vi "Treat Command.vi"(8 "error in (no error)":errorcluster, 11 "Channel in":refnum<class "Channel.lvclass">) -> (0 "error out":errorcluster, 3 "Channel out":refnum<class "Channel.lvclass">)   [LabVIEW 2018, in "Channel.lvclass"]
doc: "Treat the commando received from the control interface."
uses:
  Channel.lvclass
  Channel.lvclass/Channel.ctl
  State Machine/CCS_State Machine.lvclass
  Simulated_CCD_Camera/Simulated Camera.lvclass
  RxTx/CCS_RxTx.lvclass
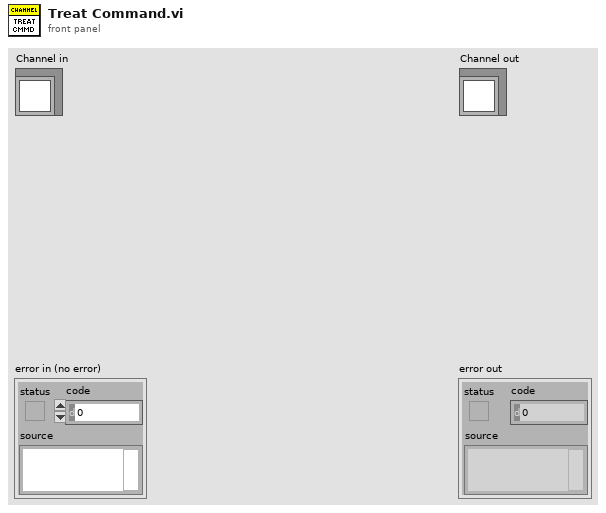
[diagram p1: front panel]
types:
  T1 = cluster{"CYCLES_DONE":u16, "LAST_IMAGE_NAME":string, "USED_DISK_SPACE":u16, "FRAMES_DONE":u16, "CCD_STATUS":string, "CURRENT_TEMPERATURE":i16, "TEMPERATURE_STATUS":string, "FRAME_EXPOSURE_TIME":sgl, "ERROR":bool, "SERIAL_NUMBER":u16, "ACQUIRING":bool, "IMAGE_INDEX":u32, "SEQS_DONE":u16}
  T2 = cluster{"COOLER_POWER_STATUS":u16, "TEMP":i32, "EXPTIME":dbl, "#FRAMES":u32, "#CYCLES":u32, "#SEQS":u32, "WAVEPLATE_POS":u16}
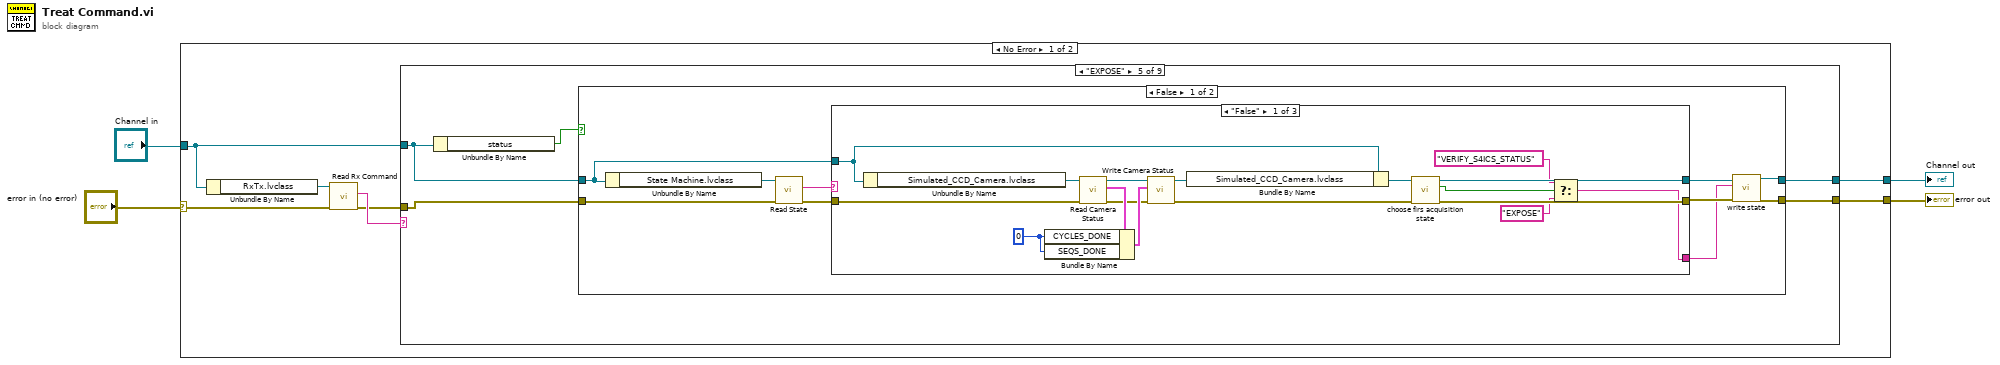
[diagram p0: block diagram]
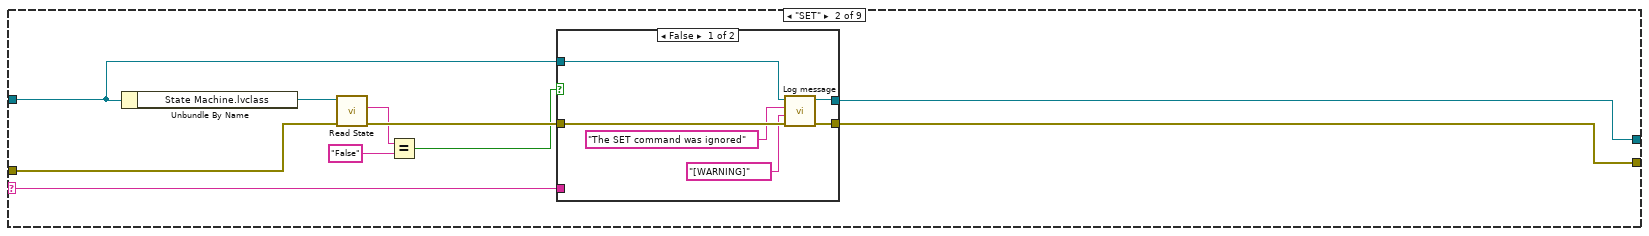
[diagram p3: hidden frame]
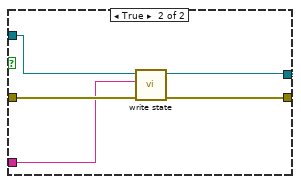
[diagram p4: hidden frame]
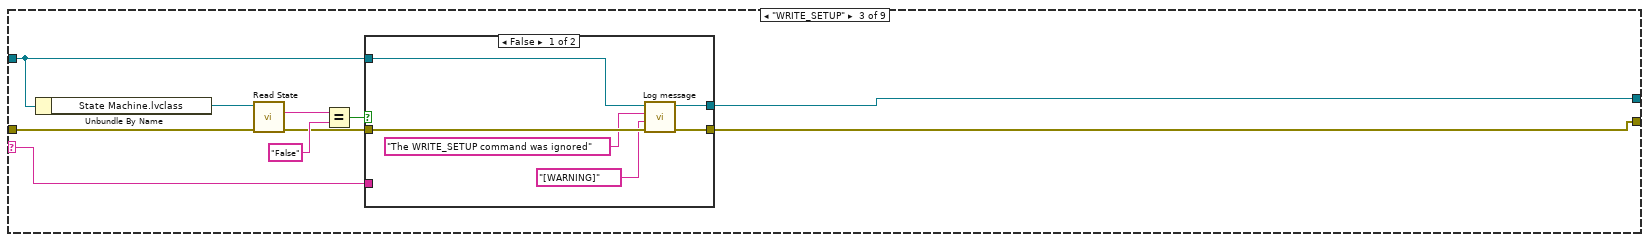
[diagram p5: hidden frame]
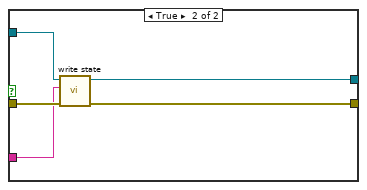
[diagram p6: hidden frame]
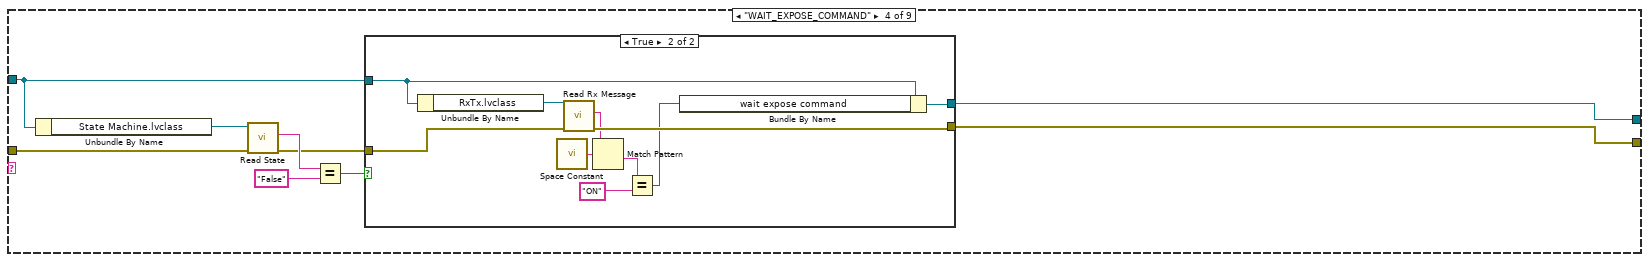
[diagram p7: hidden frame]
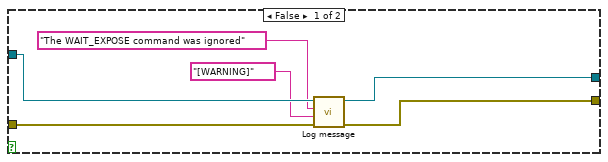
[diagram p8: hidden frame]
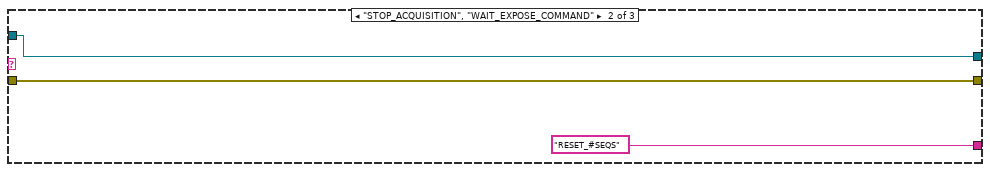
[diagram p9: hidden frame]
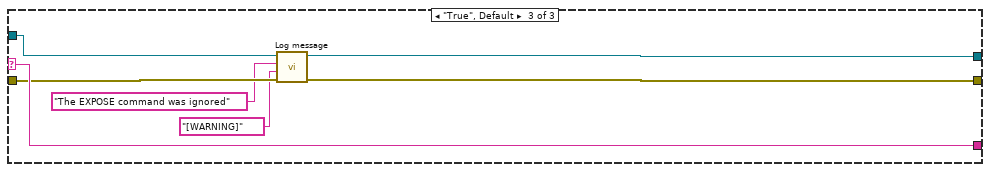
[diagram p10: hidden frame]
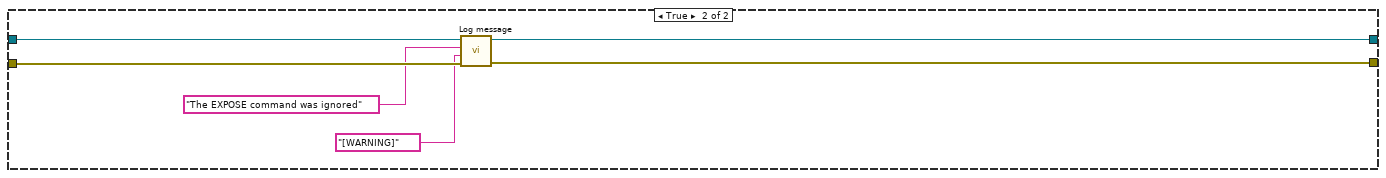
[diagram p11: hidden frame]
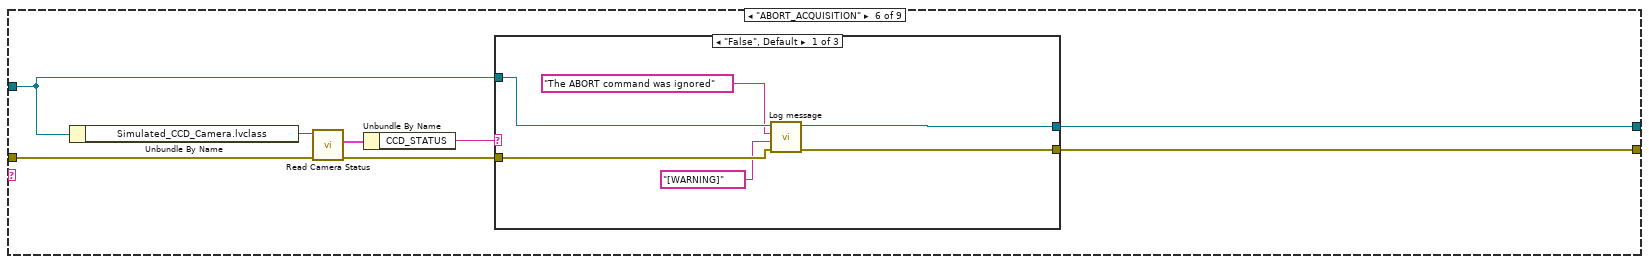
[diagram p12: hidden frame]
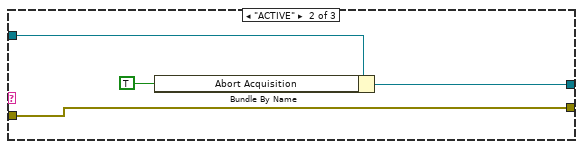
[diagram p13: hidden frame]
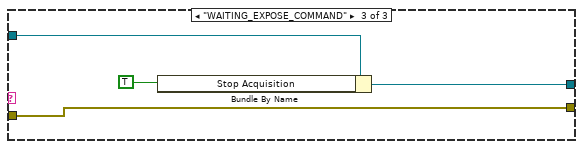
[diagram p14: hidden frame]
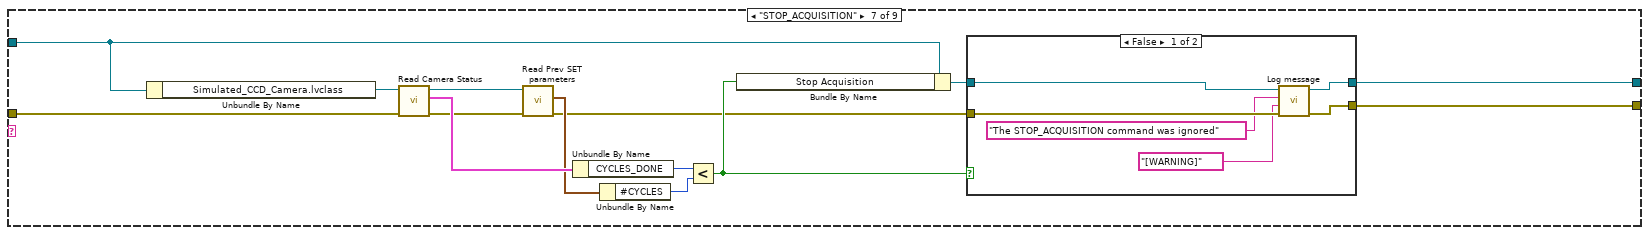
[diagram p15: hidden frame]
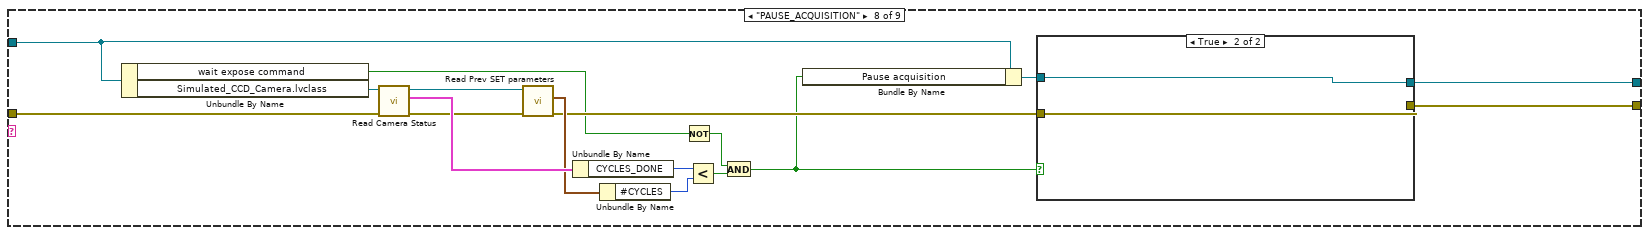
[diagram p17: hidden frame]
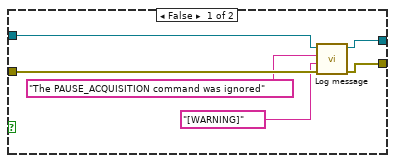
[diagram p18: hidden frame]
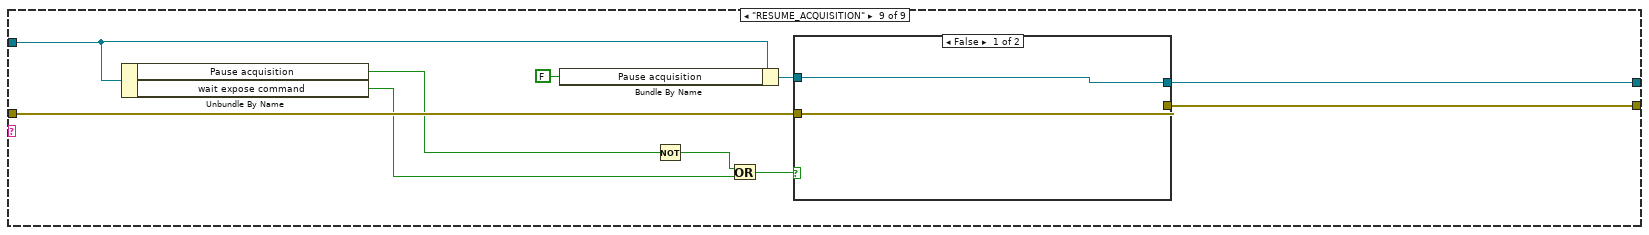
[diagram p19: hidden frame]
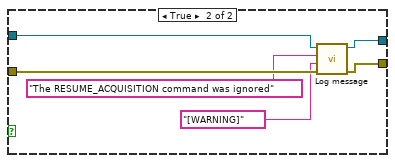
[diagram p20: hidden frame]
diagram:
  n1 = case shown="No Error" "error in (no error)" {
    selector: "error in (no error)" -> [w10 w217]
    tunnel: [w7 w217] -> w3
    tunnel: [w8 w216] -> w1
    tunnel: "Channel in" -> [w6 w216]
    frame No Error {
      n2 = Unbundle By Name(w6) -> ("RxTx.lvclass"=w11:refnum<class "CCS_RxTx.lvclass">)
      n3 = call "Read Rx Command.vi"("error in (no error)"=w10, "RxTx in"=w11) -> ("error out"=w5:errorcluster, "Rx Command"=w9:string)  [unwired: 7 in, 1 out]
      n4 = case shown="\"EXPOSE\"" w9 {
        selector: w9 -> [_ w15 w35 _ _ _ _ _ _]
        tunnel: w6 -> [w13 w17 w39 w59 w82 w136 w164 w189 w207]
        tunnel: [w13 w19 w38 w57 w84 w135 w152 w180 w205] -> w8
        tunnel: w5 -> [w12 w20 w42 w62 w83 w133 w158 w183 w206]
        tunnel: [w12 w18 w37 w56 w85 w129 w151 w179 w204] -> w7
        frame "False", Default {
        }
        frame "SET" {
          n5 = Unbundle By Name(w17) -> ("State Machine.lvclass"=w22:refnum<class "CCS_State Machine.lvclass">)
          n6 = call-dynamic "Read State.vi"("error in (no error)"=w20, "State Machine in"=w22) -> ("error out"=w23:errorcluster, "State"=w16:string)  [unwired: 7 in, 1 out]
          n7 = Equal?(x=w16, y="False") -> (x = y?=w14:bool)
          n8 = case shown="False" w14 {
            tunnel: w23 -> [w29 w31]
            tunnel: [w27 w33] -> w19
            tunnel: [w28 w32] -> w18
            tunnel: w17 -> [w26 w34]
            tunnel: w15 -> [_ w30]
            frame False {
              n9 = call "Log message.vi"("error in (no error)"=w29, "message type"="[WARNING]", "String"="The SET command was ignored", "Channel in"=w26) -> ("error out"=w28:errorcluster, "Channel out"=w27:refnum<class "Channel.lvclass">)  [unwired: 6 in]
            }
            frame True {
              n10 = call "write state.vi"("error in (no error)"=w31, "state"=w30, "Channel in"=w34) -> ("error out"=w32:errorcluster, "Channel out"=w33:refnum<class "Channel.lvclass">)  [unwired: 7 in]
            }
          }
        }
        frame "WRITE_SETUP" {
          n11 = Unbundle By Name(w39) -> ("State Machine.lvclass"=w44:refnum<class "CCS_State Machine.lvclass">)
          n12 = call-dynamic "Read State.vi"("error in (no error)"=w42, "State Machine in"=w44) -> ("error out"=w40:errorcluster, "State"=w36:string)  [unwired: 7 in, 1 out]
          n13 = Equal?(x=w36, y="False") -> (x = y?=w41:bool)
          n14 = case shown="False" w41 {
            tunnel: w40 -> [w49 w55]
            tunnel: [w47 w53] -> w38
            tunnel: [w48 w54] -> w37
            tunnel: w39 -> [w50 w52]
            tunnel: w35 -> [_ w51]
            frame False {
              n15 = call "Log message.vi"("error in (no error)"=w49, "message type"="[WARNING]", "String"="The WRITE_SETUP command was ignored", "Channel in"=w50) -> ("error out"=w48:errorcluster, "Channel out"=w47:refnum<class "Channel.lvclass">)  [unwired: 6 in]
            }
            frame True {
              n16 = call "write state.vi"("error in (no error)"=w55, "state"=w51, "Channel in"=w52) -> ("error out"=w54:errorcluster, "Channel out"=w53:refnum<class "Channel.lvclass">)  [unwired: 7 in]
            }
          }
        }
        frame "WAIT_EXPOSE_COMMAND" {
          n17 = Unbundle By Name(w59) -> ("State Machine.lvclass"=w64:refnum<class "CCS_State Machine.lvclass">)
          n18 = call-dynamic "Read State.vi"("error in (no error)"=w62, "State Machine in"=w64) -> ("error out"=w58:errorcluster, "State"=w61:string)  [unwired: 7 in, 1 out]
          n19 = Equal?(x=w61, y="False") -> (x = y?=w60:bool)
          n20 = case shown="True" w60 {
            tunnel: w59 -> [w70 w79]
            tunnel: w58 -> [w67 w80]
            tunnel: [w69 w75] -> w57
            tunnel: [w68 w76] -> w56
            frame False {
              n21 = call "Log message.vi"("error in (no error)"=w67, "message type"="[WARNING]", "String"="The WAIT_EXPOSE command was ignored", "Channel in"=w70) -> ("error out"=w68:errorcluster, "Channel out"=w69:refnum<class "Channel.lvclass">)  [unwired: 6 in]
            }
            frame True {
              n22 = Unbundle By Name(w79) -> ("RxTx.lvclass"=w78:refnum<class "CCS_RxTx.lvclass">)
              n23 = call <vilib>:"Space Constant.vi"() -> ("String"=w71:string)
              n24 = call "Read Rx Message.vi"("error in (no error)"=w80, "RxTx in"=w78) -> ("error out"=w76:errorcluster, "Rx Message"=w73:string)  [unwired: 7 in, 1 out]
              n25 = Match Pattern(string=w73, regular expression=w71) -> (after substring=w72:string)  [unwired: 1 in, 3 out]
              n26 = Equal?(x=w72, y="ON") -> (x = y?=w74:bool)
              n27 = Bundle By Name(cluster=w79, "wait expose command"=w74) -> (w75:refnum<class "Channel.lvclass">)
            }
          }
        }
        frame "EXPOSE" {
          n28 = Unbundle By Name(w82) -> ("status"=w81:bool)
          n29 = case shown="False" w81 {
            tunnel: [w88 w125] -> w85
            tunnel: w83 -> [w94 w127]
            tunnel: w82 -> [w92 w128]
            tunnel: [w89 w126] -> w84
            frame False {
              n30 = Unbundle By Name(w92) -> ("State Machine.lvclass"=w95:refnum<class "CCS_State Machine.lvclass">)
              n31 = call-dynamic "Read State.vi"("error in (no error)"=w94, "State Machine in"=w95) -> ("error out"=w91:errorcluster, "State"=w93:string)  [unwired: 7 in, 1 out]
              n32 = case shown="\"False\"" w93 {
                selector: w93 -> [_ _ w122]
                tunnel: w92 -> [w105 w114 w121]
                tunnel: w91 -> [w106 w115 w118]
                tunnel: [w102 w114 w120] -> w90
                tunnel: [w101 w115 w119] -> w87
                tunnel: [w97 "RESET_#SEQS" w122] -> w86
                frame "False" {
                  w107 = u16 0 ("CUBES_DONE")
                  n33 = Unbundle By Name(w105) -> ("Simulated_CCD_Camera.lvclass"=w108:refnum<class "Simulated Camera.lvclass">)
                  n34 = call "Read Camera Status.vi"("error in (no error)"=w106, "CCDCamera in"=w108) -> ("error out"=w109:errorcluster, "Camera Status"=w111:T1, "CCDCamera out"=w112:refnum<class "Simulated Camera.lvclass">)  [unwired: 7 in]
                  n35 = Bundle By Name(cluster=w111, "CYCLES_DONE"=w107, "SEQS_DONE"=w107) -> (w110:T1)
                  n36 = call "Write Camera Status.vi"("error in (no error)"=w109, "Camera Status"=w110, "CCDCamera in"=w112) -> ("error out"=w100:errorcluster, "CCDCamera out"=w104:refnum<class "Simulated Camera.lvclass">)  [unwired: 7 in]
                  n37 = Bundle By Name(cluster=w105, "Simulated_CCD_Camera.lvclass"=w104) -> (w103:refnum<class "Channel.lvclass">)
                  n38 = call "choose firs acquisition state.vi"("error in (no error)"=w100, "Channel in"=w103) -> ("error out"=w101:errorcluster, "verify S4ICS status"=w96:bool, "Channel out"=w102:refnum<class "Channel.lvclass">)  [unwired: 7 in]
                  n39 = Select(t="VERIFY_S4ICS_STATUS" ("x"), s=w96, f="EXPOSE" ("x")) -> (s? t:f=w97:string)
                }
                frame "STOP_ACQUISITION", "WAIT_EXPOSE_COMMAND" {
                }
                frame "True", Default {
                  n40 = call "Log message.vi"("error in (no error)"=w118, "message type"="[WARNING]", "String"="The EXPOSE command was ignored", "Channel in"=w121) -> ("error out"=w119:errorcluster, "Channel out"=w120:refnum<class "Channel.lvclass">)  [unwired: 6 in]
                }
              }
              n41 = call "write state.vi"("error in (no error)"=w87, "state"=w86, "Channel in"=w90) -> ("error out"=w88:errorcluster, "Channel out"=w89:refnum<class "Channel.lvclass">)  [unwired: 7 in]
            }
            frame True {
              n42 = call "Log message.vi"("error in (no error)"=w127, "message type"="[WARNING]", "String"="The EXPOSE command was ignored" ("Message to log"), "Channel in"=w128) -> ("error out"=w125:errorcluster, "Channel out"=w126:refnum<class "Channel.lvclass">)  [unwired: 6 in]
            }
          }
        }
        frame "ABORT_ACQUISITION" {
          n43 = Unbundle By Name(w136) -> ("Simulated_CCD_Camera.lvclass"=w132:refnum<class "Simulated Camera.lvclass">)
          n44 = call "Read Camera Status.vi"("error in (no error)"=w133, "CCDCamera in"=w132) -> ("error out"=w130:errorcluster, "Camera Status"=w134:T1)  [unwired: 7 in, 1 out]
          n45 = Unbundle By Name(w134) -> ("CCD_STATUS"=w131:string)
          n46 = case shown="\"False\", Default" w131 {
            tunnel: w136 -> [w139 w146 w150]
            tunnel: [w140 w145 w149] -> w135
            tunnel: w130 -> [w142 w143 w147]
            tunnel: [w141 w143 w147] -> w129
            frame "False", Default {
              n47 = call "Log message.vi"("error in (no error)"=w142, "message type"="[WARNING]", "String"="The ABORT command was ignored" ("Message to log"), "Channel in"=w139) -> ("error out"=w141:errorcluster, "Channel out"=w140:refnum<class "Channel.lvclass">)  [unwired: 6 in]
            }
            frame "ACTIVE" {
              n48 = Bundle By Name(cluster=w146, "Abort Acquisition"=TRUE) -> (w145:refnum<class "Channel.lvclass">)
            }
            frame "WAITING_EXPOSE_COMMAND" {
              n49 = Bundle By Name(cluster=w150, "Stop Acquisition"=TRUE ("Abort Acquisition")) -> (w149:refnum<class "Channel.lvclass">)
            }
          }
        }
        frame "STOP_ACQUISITION" {
          n50 = Unbundle By Name(w164) -> ("Simulated_CCD_Camera.lvclass"=w159:refnum<class "Simulated Camera.lvclass">)
          n51 = call "Read Camera Status.vi"("error in (no error)"=w158, "CCDCamera in"=w159) -> ("error out"=w157:errorcluster, "Camera Status"=w163:T1, "CCDCamera out"=w156:refnum<class "Simulated Camera.lvclass">)  [unwired: 7 in]
          n52 = call-dynamic "Read Prev SET parameters.vi"("error in (no error)"=w157, "Simulated_CCD_Camera in"=w156) -> ("error out"=w153:errorcluster, "Prev SET parameters"=w160:T2)  [unwired: 7 in, 1 out]
          n53 = Unbundle By Name(w163) -> ("CYCLES_DONE"=w162:u16)
          n54 = Unbundle By Name(w160) -> ("#CYCLES"=w161:u32)
          n55 = Less?(x=w162, y=w161) -> (x < y?=w154:bool)
          n56 = Bundle By Name(cluster=w164, "Stop Acquisition"=w154) -> (w155:refnum<class "Channel.lvclass">)
          n57 = case shown="False" w154 {
            tunnel: w155 -> [w170 w172]
            tunnel: w153 -> [w169 w171]
            tunnel: [w167 w172] -> w152
            tunnel: [w168 w171] -> w151
            frame False {
              n58 = call "Log message.vi"("error in (no error)"=w169, "message type"="[WARNING]", "String"="The STOP_ACQUISITION command was ignored", "Channel in"=w170) -> ("error out"=w168:errorcluster, "Channel out"=w167:refnum<class "Channel.lvclass">)  [unwired: 6 in]
            }
            frame True {
            }
          }
        }
        frame "PAUSE_ACQUISITION" {
          n59 = Unbundle By Name(w189) -> ("wait expose command"=w174:bool, "Simulated_CCD_Camera.lvclass"=w184:refnum<class "Simulated Camera.lvclass">)
          n60 = call "Read Camera Status.vi"("error in (no error)"=w183, "CCDCamera in"=w184) -> ("error out"=w182:errorcluster, "Camera Status"=w188:T1, "CCDCamera out"=w181:refnum<class "Simulated Camera.lvclass">)  [unwired: 7 in]
          n61 = call-dynamic "Read Prev SET parameters.vi"("error in (no error)"=w182, "Simulated_CCD_Camera in"=w181) -> ("error out"=w177:errorcluster, "Prev SET parameters"=w185:T2)  [unwired: 7 in, 1 out]
          n62 = Unbundle By Name(w188) -> ("CYCLES_DONE"=w187:u16)
          n63 = Unbundle By Name(w185) -> ("#CYCLES"=w186:u32)
          n64 = Not(x=w174) -> (.not. x?=w175:bool)
          n65 = Less?(x=w187, y=w186) -> (x < y?=w176:bool)
          n66 = And(x=w175, y=w176) -> (x .and. y?=w173:bool)
          n67 = Bundle By Name(cluster=w189, "Pause acquisition"=w173) -> (w178:refnum<class "Channel.lvclass">)
          n68 = case shown="True" w173 {
            tunnel: w178 -> [w195 w197]
            tunnel: w177 -> [w194 w196]
            tunnel: [w192 w197] -> w180
            tunnel: [w193 w196] -> w179
            frame False {
              n69 = call "Log message.vi"("error in (no error)"=w194, "message type"="[WARNING]", "String"="The PAUSE_ACQUISITION command was ignored", "Channel in"=w195) -> ("error out"=w193:errorcluster, "Channel out"=w192:refnum<class "Channel.lvclass">)  [unwired: 6 in]
            }
            frame True {
            }
          }
        }
        frame "RESUME_ACQUISITION" {
          n70 = Unbundle By Name(w207) -> ("Pause acquisition"=w200:bool, "wait expose command"=w201:bool)
          n71 = Bundle By Name(cluster=w207, "Pause acquisition"=FALSE ("Acquisition control.Pause acquisition")) -> (w203:refnum<class "Channel.lvclass">)
          n72 = Not(x=w200) -> (.not. x?=w199:bool)
          n73 = Or(x=w199, y=w201) -> (x .or. y?=w198:bool)
          n74 = case shown="False" w198 {
            tunnel: w203 -> [w209 w215]
            tunnel: w206 -> [w208 w214]
            tunnel: [w209 w212] -> w205
            tunnel: [w208 w213] -> w204
            frame False {
            }
            frame True {
              n75 = call "Log message.vi"("error in (no error)"=w214, "message type"="[WARNING]", "String"="The RESUME_ACQUISITION command was ignored", "Channel in"=w215) -> ("error out"=w213:errorcluster, "Channel out"=w212:refnum<class "Channel.lvclass">)  [unwired: 6 in]
            }
          }
        }
      }
    }
    frame Error {
    }
  }
  "error out" <- w3
  "Channel out" <- w1
